vi "ArmUPandDOWN.vi"(0 "Lower Limit":string="My DI RefNum", 1 "Arm Value":dbl, 5 "Upper Limit":string="My DI RefNum", 7 "Arm":string="My Motor RefNum", 9 "Override":bool, 11 "Error In":errorcluster) -> (4 "UpperLimit":bool, 6 "LowerLimit":bool, 15 "Error Out":errorcluster)   [LabVIEW 2014]
panel:
  out "Arm Power":dbl
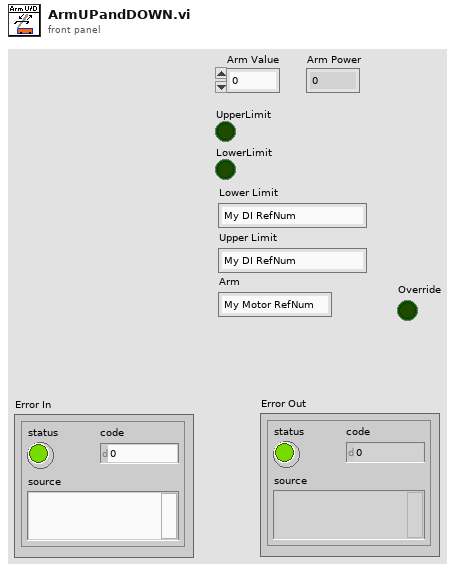
[diagram p1: front panel]
types:
  T1 = typedef "WPI_DigitalInputDevRef.ctl" = cluster{"DevStatus":errorcluster, "DIO Channel":T2, "Controller":T3}
  T2 = typedef "FPGA_DIOChannel.ctl" = enum8{"DIO 0", "DIO 1", "DIO 2", "DIO 3", "DIO 4", "DIO 5", "DIO 6", "DIO 7", "DIO 8", "DIO 9", "DIO MXP 0", "DIO MXP 1", "DIO MXP 2", "DIO MXP 3", "DIO MXP 4", "DIO MXP 5", "DIO MXP 6", "DIO MXP 7", "DIO MXP 8", "DIO MXP 9", "DIO MXP 10", "DIO MXP 11", "DIO MXP 12", "DIO MXP 13", "DIO MXP 14", "DIO MXP 15", "Invalid"}
  T3 = typedef "FPGA_TypedefDigitalModule.ctl" = enum16{"Controller 1"}
  T4 = typedef "WPI_MotorControlDeviceRef.ctl" = cluster{"DeviceStatus":errorcluster, "Type":T5, "PWM":cluster{"Controller":T3, "PWM Channel":T6, "DeadBand":T7}, "CAN":cluster{"Device Number":u8, "Control Mode":T8, "Semaphore":T9, "Max Vout":dbl, "TalonSRX Control Mode":T10}, "Invert":bool, "TransformRef":T11, "InvTransformRef":T11}
  T5 = typedef "WPI_MotorControlType.ctl" = enum16{"PWM", "CAN", "CANTalonSRX"}
  T6 = typedef "FPGA_DIOPWMChannel.ctl" = enum8{"PWM 0", "PWM 1", "PWM 2", "PWM 3", "PWM 4", "PWM 5", "PWM 6", "PWM 7", "PWM 8", "PWM 9", "PWM MXP 0", "PWM MXP 1", "PWM MXP 2", "PWM MXP 3", "PWM MXP 4", "PWM MXP 5", "PWM MXP 6", "PWM MXP 7", "PWM MXP 8", "PWM MXP 9", "Invalid"}
  T7 = typedef "WPI_PWMDeadband.ctl" = cluster{"Name":string, "maxPositivePwm":i32, "minPositivePwm":i32, "centerPwm":i32, "maxNegativePwm":i32, "minNegativePwm":i32, "angularRange":u16}
  T8 = typedef "WPI_CANJaguar_ControlMode.ctl" = enum8{"Percent VBus", "Current", "Speed", "Position", "Voltage"}
  T9 = typedef "Semaphore RefNum" = refnum<k1>
  T10 = typedef "WPI_CANTalonSRX_APIControlMode.ctl" = enum8{"Percent VBus", "Speed", "Position", "Slave", "Unchanged / Invalid"}
  T11 = typedef "WPI_PWMTransform_ConPane.ctl" = refnum<vi>
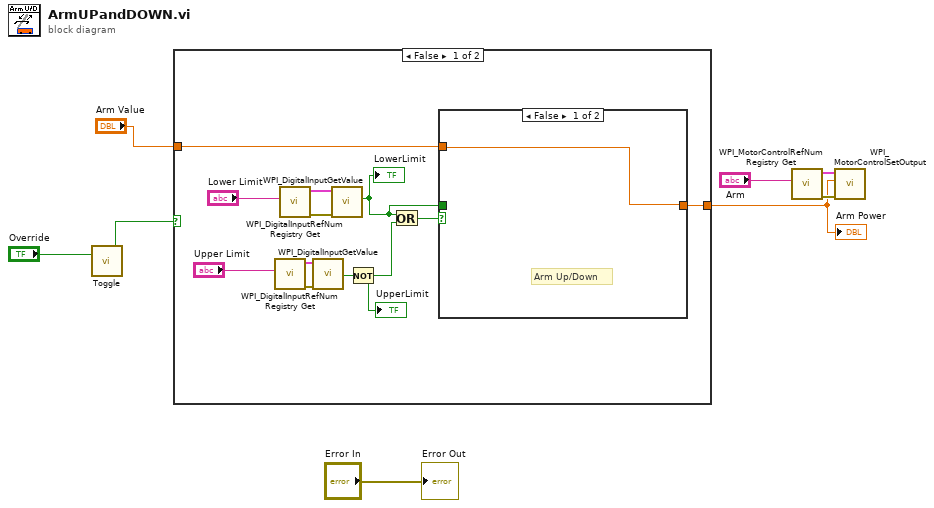
[diagram p0: block diagram]
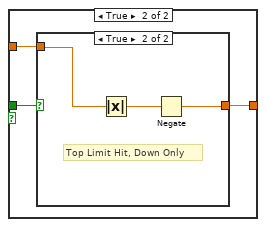
[diagram p2: hidden frame]
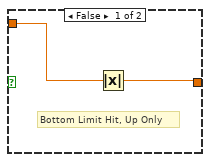
[diagram p3: hidden frame]
diagram:
  n1 = call "Toggle.vi"("Input"="Override") -> ("Output"=w2:bool)
  n2 = case shown="False" w2 {
    tunnel: [w15 w30] -> w6
    tunnel: "Arm Value" -> [w11 w30]
    frame False {
      n3 = call <vilib>:"WPI_DigitalInputRefNum Registry Get.vi"("refnum name"="Upper Limit") -> ("error out"=w17:errorcluster, "DigitalInputDevRef"=w18:T1)  [unwired: 9 in]
      n4 = call <vilib>:"WPI_DigitalInputRefNum Registry Get.vi"("refnum name"="Lower Limit") -> ("error out"=w20:errorcluster, "DigitalInputDevRef"=w19:T1)  [unwired: 9 in]
      n5 = call <vilib>:"WPI_DigitalInputGetValue.vi"("error in (no error)"=w17, "DigitalInputDevRef"=w18) -> ("Value"=w9:bool)  [unwired: 7 in, 2 out]
      n6 = call <vilib>:"WPI_DigitalInputGetValue.vi"("error in (no error)"=w20, "DigitalInputDevRef"=w19) -> ("Value"=w16:bool)  [unwired: 7 in, 2 out]
      "LowerLimit" <- w16
      n7 = Not(x=w9) -> (.not. x?=w10:bool)
      "UpperLimit" <- w10
      n8 = Or(x=w16, y=w10) -> (x .or. y?=w14:bool)
      n9 = case shown="False" w14 {
        tunnel: [w21 w23] -> w15
        tunnel: w16 -> [_ w24]
        tunnel: w11 -> [w21 w22]
        frame False {
          # "Arm Up/Down"
        }
        frame True {
          n10 = case shown="True" w24 {
            tunnel: [w26 w29] -> w23
            tunnel: w22 -> [w25 w27]
            frame False {
              # "Bottom Limit Hit, Up Only"
              n11 = Absolute Value(x=w25) -> (abs(x)=w26:dbl)
            }
            frame True {
              # "Top Limit Hit, Down Only"
              n12 = Absolute Value(x=w27) -> (abs(x)=w28:dbl)
              n13 = Negate(x=w28) -> (-x=w29:dbl)
            }
          }
        }
      }
    }
    frame True {
    }
  }
  "Arm Power" <- w6
  n14 = call <vilib>:"WPI_MotorControlRefNum Registry Get.vi"("refnum name"="Arm") -> ("error out"=w7:errorcluster, "MotorControlDevRef"=w8:T4)  [unwired: 9 in]
  n15 = call <vilib>:"WPI_MotorControlSetOutput.vi"("error in (no error)"=w7, "Output"=w6, "MotorControlDevRef"=w8) -> ()  [unwired: 6 in, 3 out]
  "Error Out" <- "Error In"
